vi "gradual_motorset_diag.vi"(7 "Initial Voltage (V)":dbl, 8 "error in (no error)":errorcluster, 9 "Steps":dbl, 10 "Next Voltage (V)":dbl, 11 "Physical Channel":tag="Dev1/ao0") -> (0 "error out":errorcluster)   [LabVIEW 2013]
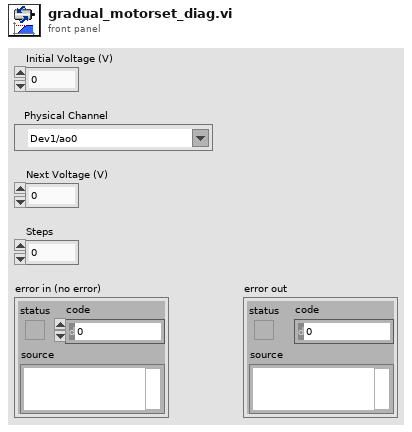
[diagram p1: front panel]
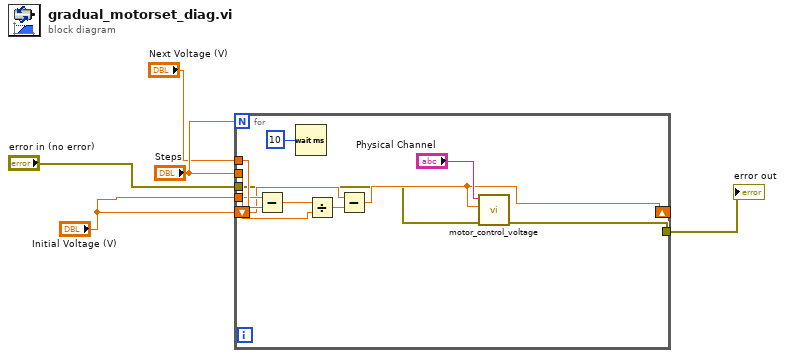
[diagram p0: block diagram]
diagram:
  n1 = for {
    N: "Steps" -> [_]
    tunnel: "error in (no error)" -> [w6]
    tunnel: "Initial Voltage (V)" -> [w12]
    tunnel: "Next Voltage (V)" -> [w15]
    tunnel: "Steps" -> [w13]
    shift-right: [w8] -> _
    shift-left: "Initial Voltage (V)" -> [w11]
    tunnel: [w9] -> w5
    n2 = Subtract(x=w12, y=w15) -> (x-y=w16:dbl)
    n3 = Wait (ms)(milliseconds to wait=u32 10) -> ()  [unwired: 1 out]
    n4 = Divide(x=w16, y=w13) -> (x/y=w14:dbl)
    n5 = Subtract(x=w11, y=w14) -> (x-y=w8:dbl)
    n6 = call "motor_control_voltage.vi"("Error In"=w6, "Numeric"=w8, "Physical Channel"="Physical Channel") -> ("error out"=w9:errorcluster)  [unwired: 8 in]
  }
  "error out" <- w5
